vi "Define String.vi"(7 "add ifndef/endif (F)":bool, 9 "Value":string, 10 "Name":string, 11 "String in":string) -> (3 "String out":string)   [LabVIEW 2014, in "C Header Generator.lvlib"]
uses:
  C Header Generator.lvlib
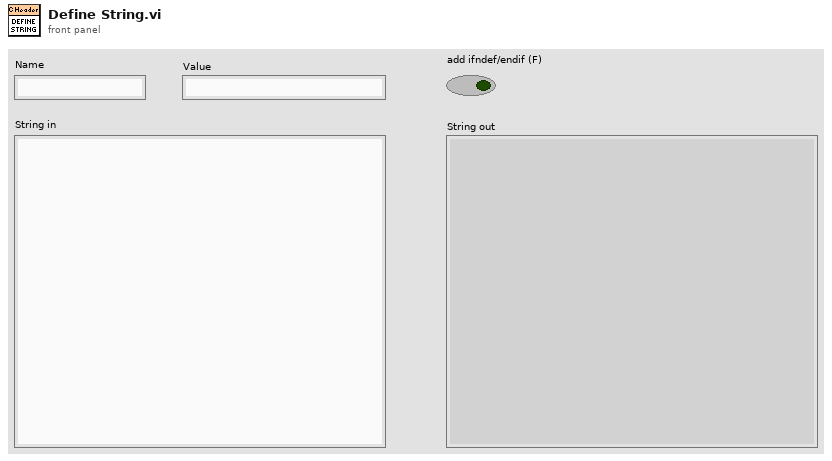
[diagram p1: front panel]
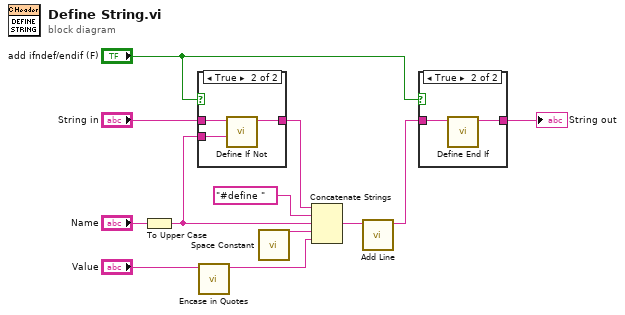
[diagram p0: block diagram]
diagram:
  n1 = To Upper Case(1:"Name") -> (0:w1:string)
  n2 = case shown="True" "add ifndef/endif (F)" {
    tunnel: "String in" -> [w13 w16]
    tunnel: [w13 w15] -> w6
    tunnel: w1 -> [_ w14]
    frame False {
    }
    frame True {
      n3 = call "Define If Not.vi"("token string"=w14, "String in"=w16) -> ("String out"=w15:string)  [unwired: 9 in]
    }
  }
  n4 = call "Encase in Quotes.vi"("String in"="Value") -> ("String out"=w8:string)  [unwired: 10 in]
  n5 = call <vilib>:"Space Constant.vi"() -> ("String"=w11:string)
  n6 = Concatenate Strings(w6, "#define ", w1, w11, w8) -> (w10:string)
  n7 = call "Add Line.vi"("String in"=w10) -> ("String out"=w3:string)  [unwired: 10 in]
  n8 = case shown="True" "add ifndef/endif (F)" {
    tunnel: w3 -> [w17 w19]
    tunnel: [w17 w18] -> w4
    frame False {
    }
    frame True {
      n9 = call "Define End If.vi"("String in"=w19) -> ("String out"=w18:string)  [unwired: 10 in]
    }
  }
  "String out" <- w4
